vi "Nov_30 - Ramp Mode.vi"() -> ()   [LabVIEW 2020]
uses:
  <vilib>/Utility/error.llb/DialogType.ctl
  <vilib>/Analysis/3filter.llb/Filter Passband Type.ctl
  <vilib>/DAQmx/read.llb/DAQmx Read (Analog 1D DBL NChan 1Samp).vi
  <vilib>/DAQmx/create/channels.llb/DAQmx Create Channel (AI-Voltage-Basic).vi
  <vilib>/DAQmx/configure/timing.llb/DAQmx Timing (Sample Clock).vi
  <vilib>/DAQmx/miscellaneous.llb/DAQmx Fill In Error Info.vi
  <vilib>/Analysis/3filter.llb/Butterworth Filter (DBL).vi
  <vilib>/Utility/file.llb/Write Delimited Spreadsheet (string).vi
  <vilib>/Utility/file.llb/Write Delimited Spreadsheet (DBL).vi
  <vilib>/Analysis/NI_AALBase.lvlib
panel:
  out "Swing ON time":dbl
  out "Register Time":bool
  out "Swing Start Time":dbl
  out "Pre-Tension Load (N)":dbl
  out "Time To Peak (ms)":dbl
  out "Peak Value (ms)":dbl=2.0
  out "Square Wave Amp Target (N)":dbl=2.0
  in  "Auto Mode":string(combo)
  out "Release":bool
  out "Pull":bool
  in  "Working Mode":string(combo)
  out "Load Cell":dbl
  in  "Pull CMD":bool
  in  "Release CMD":bool
  out "Load Cell":dynamicdata(graph)
  in  "Motor Torque":dbl(slide) scale=0.0..5.0
  out "Swing (Consumer Loop)":bool
  in  "Master Stop":bool
  out "Consumer Loop Speed (ms)":u32
  out "Producer Loop Speed (ms)":u32
  out "Swing":bool
  out "Force Plate":dynamicdata(graph)
  out "Accelerometers":dynamicdata(graph)
  out "Enlapsed Time (sec)":dbl
  # "Motor Control"
  # "Manual"
  # "Automatic"
  # "Square"
  # "Ramp"
  # "Indicators"
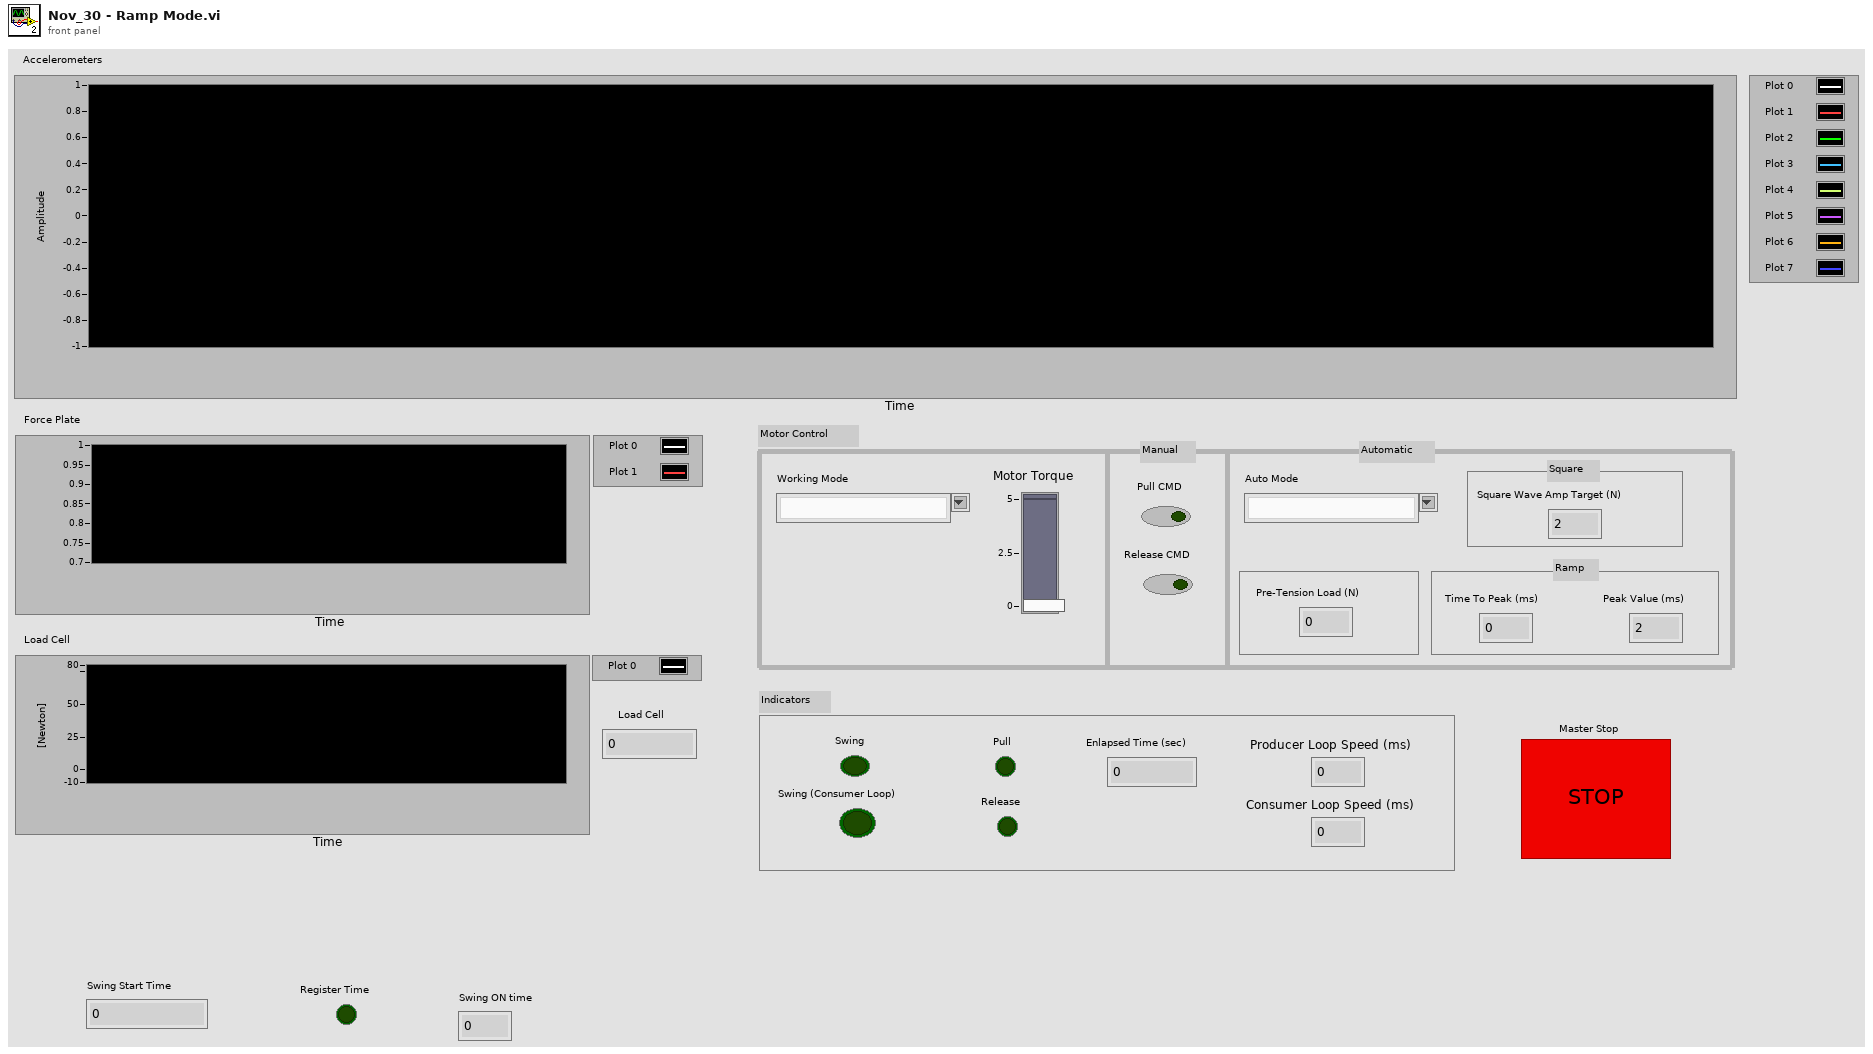
[diagram p1: front panel]
types:
  T1 = typedef "DialogType.ctl" = u16
  T2 = typedef "NI_AALBase.lvlib/Filter Passband Type.ctl" = enum32{"Lowpass", "Highpass", "Bandpass", "Bandstop"}
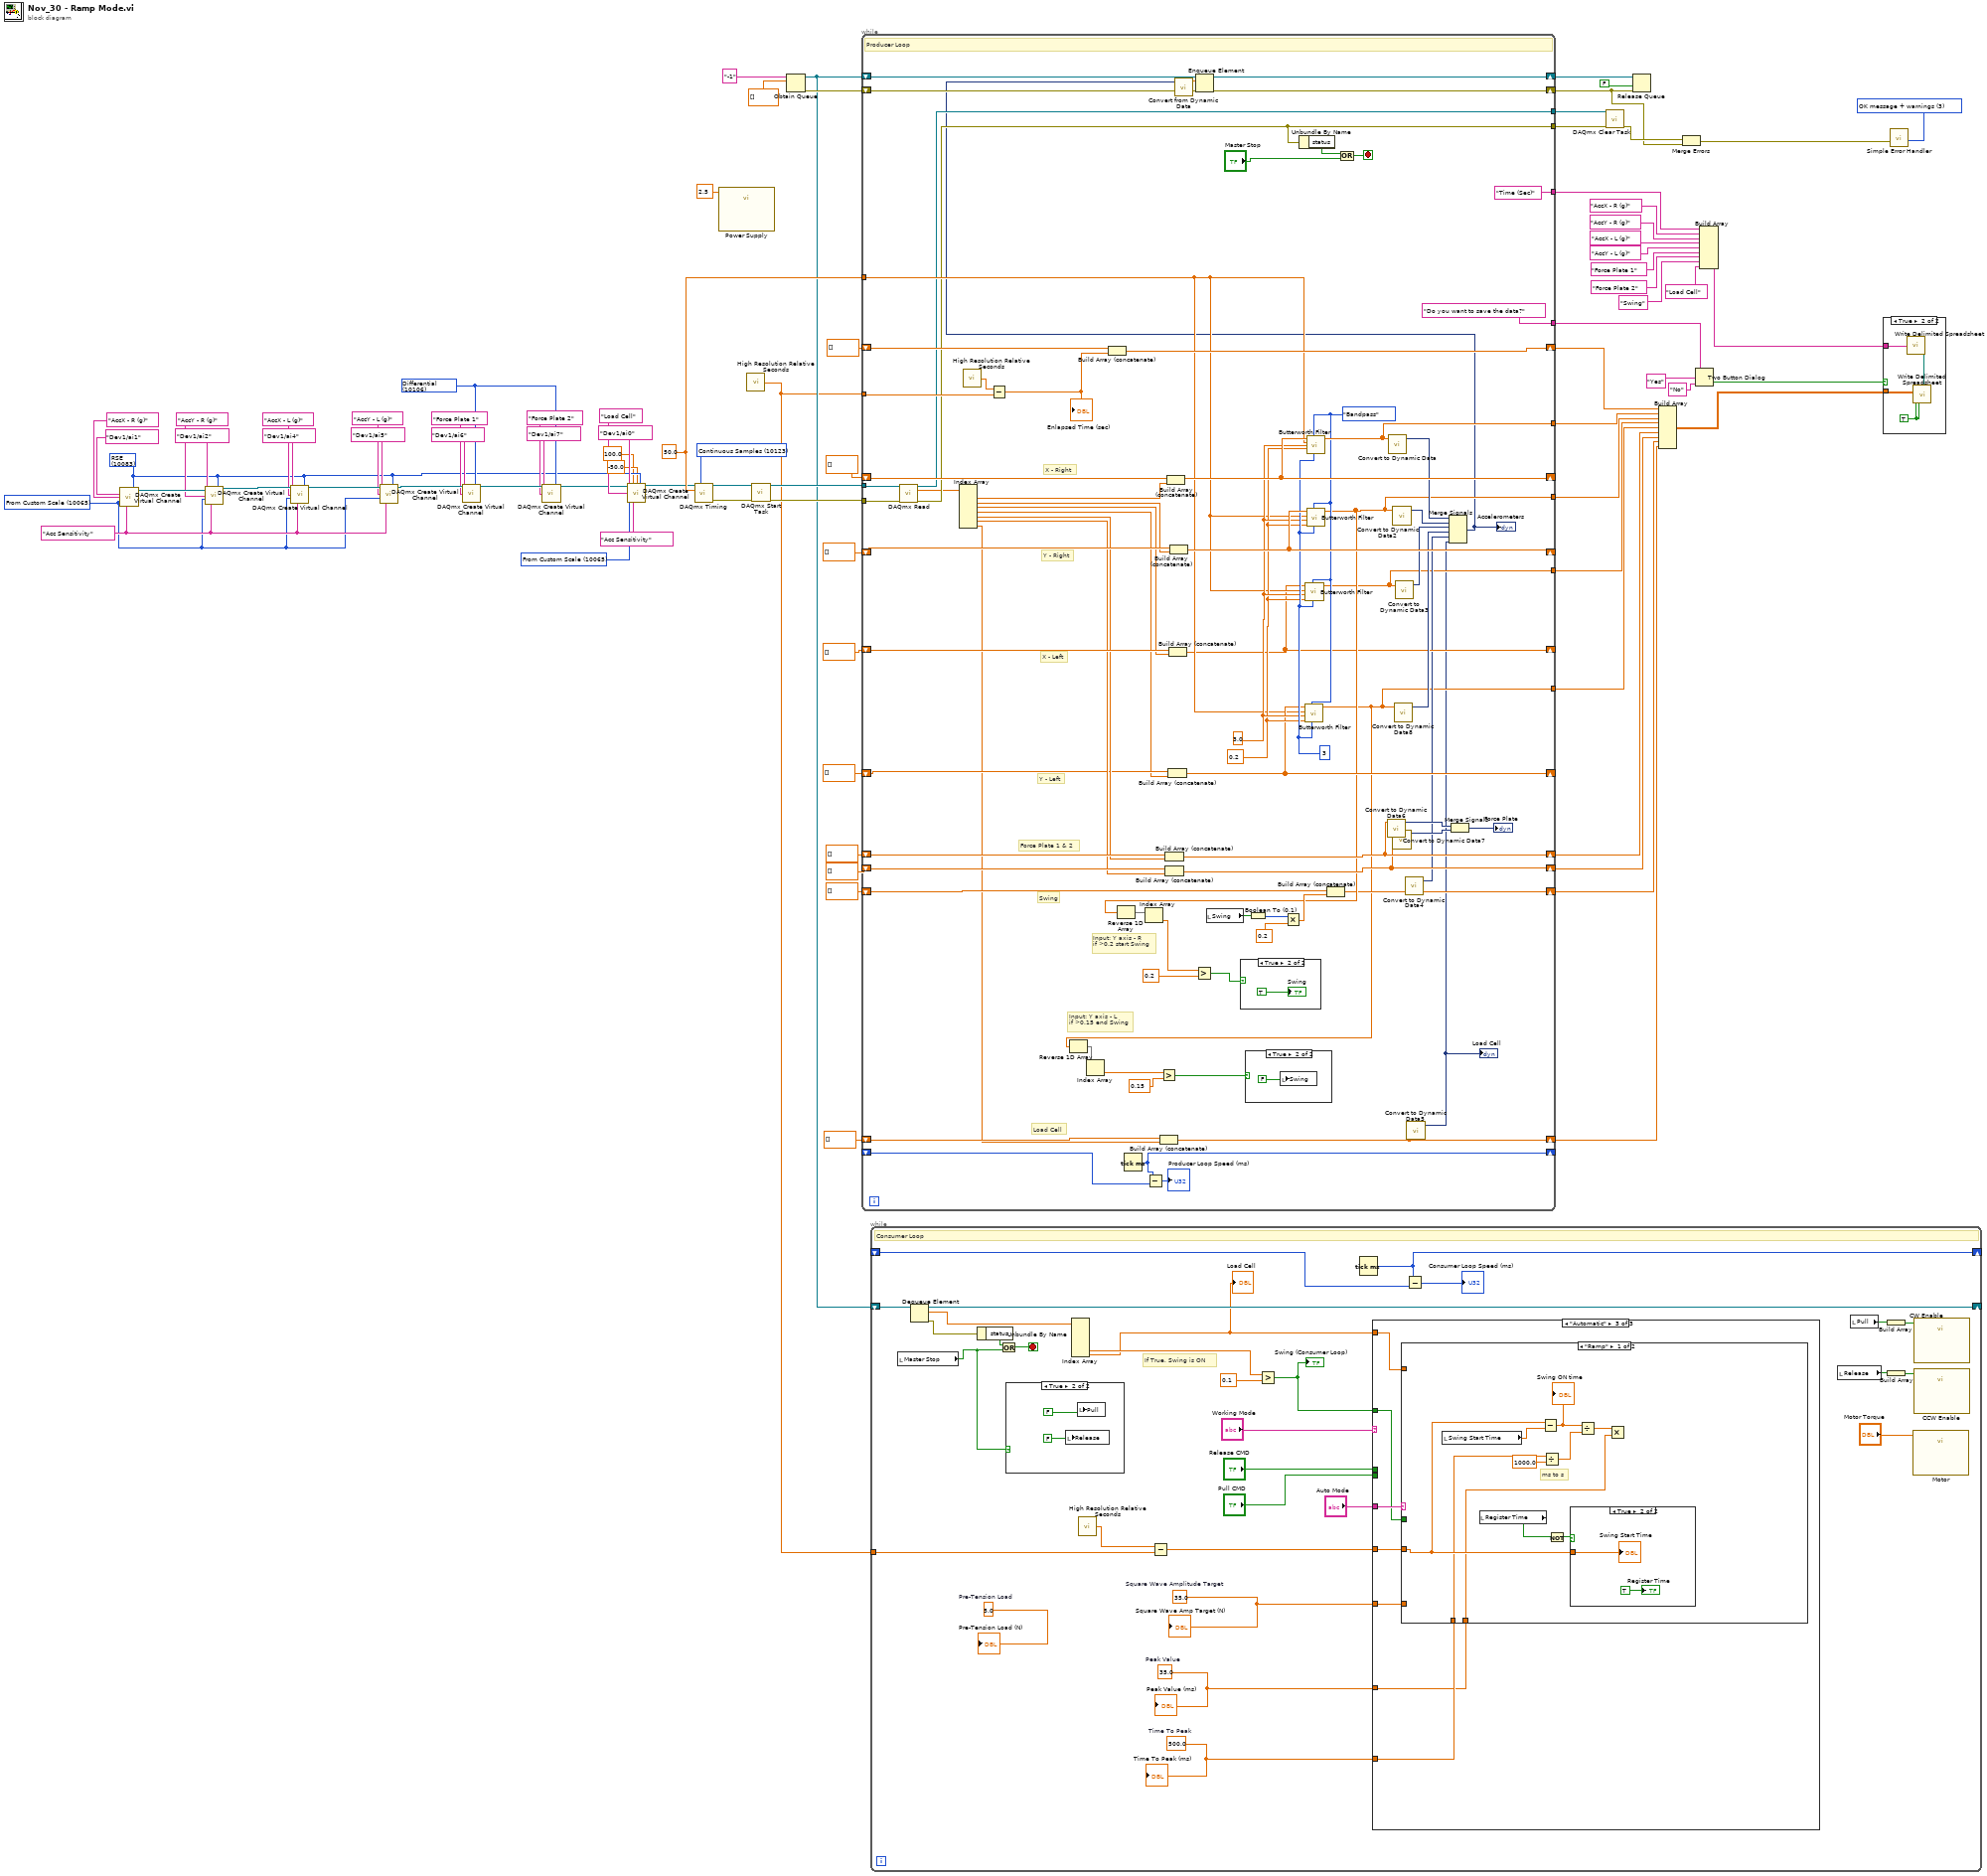
[diagram p0: block diagram]
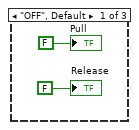
[diagram p3: hidden frame]
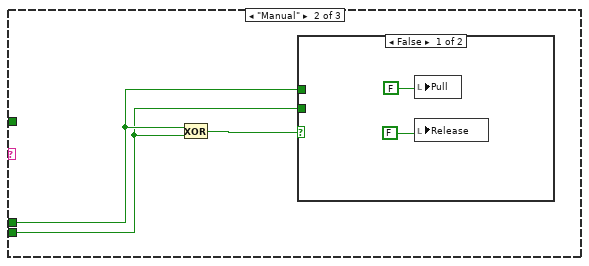
[diagram p4: hidden frame]
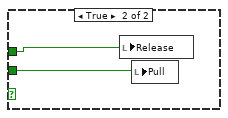
[diagram p5: hidden frame]
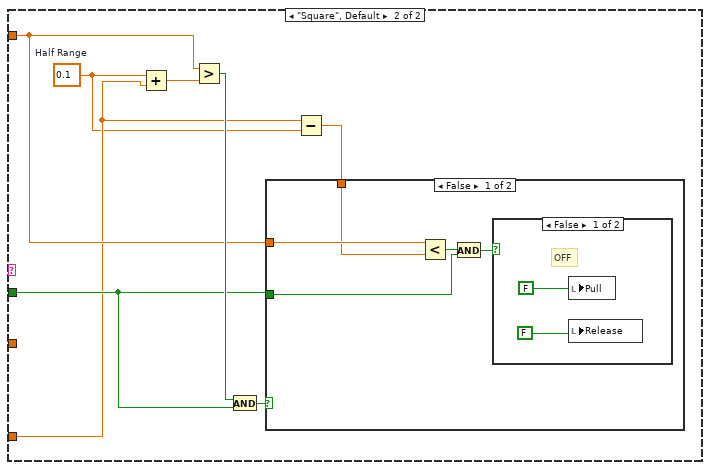
[diagram p7: hidden frame]
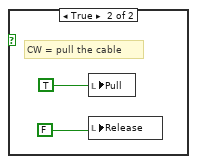
[diagram p8: hidden frame]
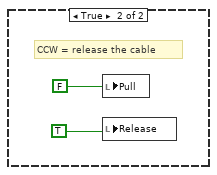
[diagram p9: hidden frame]
diagram:
  w4 = 10065 items=["Volts"=10348, "From Custom Scale"=10065] ("units")
  w20 = T1 3 items=["no dialog", "OK message", "continue or stop message", "OK message + warnings", "continue/stop + warnings"] ("type of dialog (OK msg:1)")
  w9 = 10065 items=["Volts"=10348, "From Custom Scale"=10065] ("units")
  w10 = tag "Acc Sensitivity" ("custom scale name")
  w30 = 10106 items=["Default"=-1, "RSE"=10083, "NRSE"=10078, "Differential"=10106, "Pseudodifferential"=12529] ("input terminal configuration")
  w52 = 10123 items=["Finite Samples"=10178, "Continuous Samples"=10123, "Hardware Timed Single Point"=12522] ("sample mode")
  w47 = 50.0 ("rate")
  w13 = 10083 items=["Default"=-1, "RSE"=10083, "NRSE"=10078, "Differential"=10106, "Pseudodifferential"=12529] ("input terminal configuration")
  n1 = call-poly <vilib>:"DAQmx Create Virtual Channel.vi"("input terminal configuration"=w13, "physical channels"=tag "Dev1/ai1" ("Physical channels"), "name to assign"="AccX - R (g)", "units"=w9, "custom scale name"=w10) -> ("task out"=w46:refnum<k21>)  [unwired: 9 in, 1 out]
  n2 = call-poly <vilib>:"DAQmx Create Virtual Channel.vi"("task in"=w46, "input terminal configuration"=w13, "physical channels"=tag "Dev1/ai2", "name to assign"="AccY - R (g)", "units"=w9, "custom scale name"=w10) -> ("task out"=w45:refnum<k21>)  [unwired: 8 in, 1 out]
  n3 = call-poly <vilib>:"DAQmx Create Virtual Channel.vi"("task in"=w45, "input terminal configuration"=w13, "physical channels"=tag "Dev1/ai4", "name to assign"="AccX - L (g)", "units"=w9, "custom scale name"=w10) -> ("task out"=w44:refnum<k21>)  [unwired: 8 in, 1 out]
  n4 = call-poly <vilib>:"DAQmx Create Virtual Channel.vi"("task in"=w44, "input terminal configuration"=w13, "physical channels"=tag "Dev1/ai5", "name to assign"="AccY - L (g)", "units"=w9, "custom scale name"=w10) -> ("task out"=w43:refnum<k21>)  [unwired: 8 in, 1 out]
  n5 = call-poly <vilib>:"DAQmx Create Virtual Channel.vi"("task in"=w43, "input terminal configuration"=w30, "physical channels"=tag "Dev1/ai6", "name to assign"="Force Plate 1" ("element")) -> ("task out"=w37:refnum<k21>)  [unwired: 10 in, 1 out]
  n6 = call-poly <vilib>:"DAQmx Create Virtual Channel.vi"("task in"=w37, "input terminal configuration"=w30, "physical channels"=tag "Dev1/ai7", "name to assign"="Force Plate 2" ("element")) -> ("task out"=w12:refnum<k21>)  [unwired: 10 in, 1 out]
  n7 = call-poly <vilib>:"DAQmx Create Virtual Channel.vi"("task in"=w12, "maximum value"=100.0, "minimum value"=-50.0, "input terminal configuration"=w13, "physical channels"=tag "Dev1/ai0", "name to assign"="Load Cell", "units"=w4, "custom scale name"=tag "Acc Sensitivity") -> ("task out"=w11:refnum<k21>)  [unwired: 6 in, 1 out]
  n8 = call-poly <vilib>:"DAQmx Timing.vi"("task/channels in"=w11, "sample mode"=w52, "rate"=w47) -> ("task out"=w51:refnum<k21>, "error out"=w50:errorcluster)  [unwired: 11 in]
  n9 = call "Power Supply"("data"=2.5) -> ()  [unwired: 17 in, 2 out]
  n10 = call <vilib>:"High Resolution Relative Seconds.vi"() -> ("relative seconds"=w1:dbl)
  n11 = call <vilib>:"DAQmx Start Task.vi"("task/channels in"=w51, "error in"=w50) -> ("task out"=w49:refnum<k21>, "error out"=w48:errorcluster)  [unwired: 12 in]
  n12 = Obtain Queue(name (unnamed)="-1", element data type=dbl[] []) -> (queue out=w16:refnum<queue>, error out=w25:errorcluster)  [unwired: 3 in, 1 out]
  n13 = while {
    tunnel: w49 -> [w159]
    tunnel: w48 -> [w158]
    tunnel: w1 -> [w156]
    shift-right: [w140] -> w80
    shift-left: dbl[] [] -> [w154]
    shift-right: [w144] -> _
    shift-left: dbl[] [] -> [w153]
    shift-right: [w143] -> _
    shift-left: dbl[] [] -> [w152]
    tunnel: ["Time (Sec)"] -> w55
    tunnel: ["Do you want to save the data?" ("message")] -> w72
    shift-right: [w104] -> w59
    shift-left: dbl[] [] -> [w149]
    shift-right: [w105] -> _
    shift-left: dbl[] [] -> [w141]
    shift-right: [w130] -> w57
    shift-left: dbl[] [] -> [w133]
    shift-right: [w128] -> w58
    shift-left: dbl[] [] -> [w132]
    tunnel: [w126] -> w62
    tunnel: [w108] -> w61
    tunnel: [w100] -> w60
    shift-right: [w119] -> _
    shift-left: dbl[] [] -> [w118]
    tunnel: [w99] -> w56
    tunnel: w47 -> [w116]
    shift-right: [w110] -> _
    shift-left: _ -> [w109]
    shift-right: [w93] -> w24
    shift-left: w16 -> [w94]
    shift-right: [w91] -> w17
    shift-left: w25 -> [w92]
    tunnel: [w98] -> w22
    tunnel: [w95] -> w21
    shift-right: [w86] -> w7
    shift-left: dbl[] [] -> [w85]
    stop <- w96 stop-if-true
    w123 = 3 ("order")
    w121 = 0.2 ("low cutoff freq: fl")
    w122 = 3.0 ("high cutoff freq: fh")
    w117 = Filter_Passband_Type."Bandpass" ("filter type")
    # "X - Right"
    # "Y - Right"
    # "X - Left"
    # "Y - Left"
    # "Force Plate 1 & 2"
    # "Swing"
    # "Load Cell"
    # "Input: Y axis - L\nif >0.15 end Swing"
    # "Input: Y axis - R\nif >0.2 start Swing"
    # "Producer Loop"
    n14 = call-poly <vilib>:"DAQmx Read.vi"("task/channels in"=w159, "error in"=w158) -> ("task out"=w98:refnum<k21>, "data"=w90:dbl[], "error out"=w95:errorcluster)  [unwired: 11 in]
    n15 = Index Array(array=w90) -> (element #1=w115:dbl, element #2=w114:dbl, element #3=w113:dbl, element #4=w112:dbl, element #5=w124:dbl, element #6=w125:dbl, element #7=w84:dbl)  [unwired: 7 in]
    n16 = call <vilib>:"High Resolution Relative Seconds.vi"() -> ("relative seconds"=w157:dbl)
    n17 = Subtract(x=w157, y=w156) -> (x-y=w155:dbl)
    "Enlapsed Time (sec)" <- w155
    n18 = Build Array (concatenate)(w154, w155) -> (w140:dbl[])
    n19 = Tick Count (ms)() -> (millisecond timer value=w110:u32)
    n20 = Subtract(x=w110, y=w109) -> (x-y=→"Producer Loop Speed (ms)":u32)
    n21 = Build Array (concatenate)(w85, w84) -> (w86:dbl[])
    n22 = Build Array (concatenate)(w133, w124) -> (w130:dbl[])
    n23 = Build Array (concatenate)(w132, w125) -> (w128:dbl[])
    n24 = Build Array (concatenate)(w153, w115) -> (w144:dbl[])
    n25 = Build Array (concatenate)(w118, w112) -> (w119:dbl[])
    n26 = Build Array (concatenate)(w141, w113) -> (w105:dbl[])
    n27 = Build Array (concatenate)(w152, w114) -> (w143:dbl[])
    n28 = local read "Swing"() -> (w142:bool)
    n29 = Boolean To (0,1)(Boolean=w142) -> (0, 1=w147:i16)
    n30 = Multiply(x=w147, y=0.2) -> (x*y=w148:dbl)
    n31 = Unbundle By Name(w95) -> ("status"=w97:bool)
    n32 = call-poly <vilib>:"Butterworth Filter.vi"("order"=w123, "filter type"=w117, "low cutoff freq: fl"=w121, "high cutoff freq: fh"=w122, "sampling freq: fs"=w116, "X"=w119) -> ("Filtered X"=w99:dbl[])  [unwired: 2 in, 1 out]
    n33 = Reverse 1D Array(array=w99) -> (reversed array=w135:dbl[])
    n34 = Index Array(array=w135) -> (element=w134:dbl)  [unwired: 1 in]
    n35 = Greater?(x=w134, y=0.15) -> (0:w102:bool)
    n36 = case shown="True" w102 {
      frame False {
      }
      frame True {
        n37 = local write "Swing"(FALSE) -> ()
      }
    }
    n38 = call-poly <vilib>:"Butterworth Filter.vi"("order"=w123, "filter type"=w117, "low cutoff freq: fl"=w121, "high cutoff freq: fh"=w122, "sampling freq: fs"=w116, "X"=w105) -> ("Filtered X"=w100:dbl[])  [unwired: 2 in, 1 out]
    n39 = call-poly <vilib>:"Butterworth Filter.vi"("order"=w123, "filter type"=w117, "low cutoff freq: fl"=w121, "high cutoff freq: fh"=w122, "sampling freq: fs"=w116, "X"=w144) -> ("Filtered X"=w126:dbl[])  [unwired: 2 in, 1 out]
    n40 = call-poly <vilib>:"Butterworth Filter.vi"("order"=w123, "filter type"=w117, "low cutoff freq: fl"=w121, "high cutoff freq: fh"=w122, "sampling freq: fs"=w116, "X"=w143) -> ("Filtered X"=w108:dbl[])  [unwired: 2 in, 1 out]
    n41 = Reverse 1D Array(array=w108) -> (reversed array=w145:dbl[])
    n42 = Index Array(array=w145) -> (element=w107:dbl)  [unwired: 1 in]
    n43 = Greater?(x=w107, y=0.2) -> (0:w101:bool)
    n44 = case shown="True" w101 {
      frame False {
      }
      frame True {
        "Swing" <- TRUE
      }
    }
    n45 = Build Array (concatenate)(w149, w148) -> (w104:dbl[])
    n46 = Or(x=w97, y="Master Stop") -> (x .or. y?=w96:bool)
    n47 = call "Convert to Dynamic Data6"("Array"=w130) -> ("Dynamic Data Type"=w129:dynamicdata)  [unwired: 3 in]
    n48 = call "Convert to Dynamic Data"("Array"=w126) -> ("Dynamic Data Type"=w139:dynamicdata)  [unwired: 3 in]
    n49 = call "Convert to Dynamic Data2"("Array"=w108) -> ("Dynamic Data Type"=w138:dynamicdata)  [unwired: 3 in]
    n50 = call "Convert to Dynamic Data7"("Array"=w128) -> ("Dynamic Data Type"=w127:dynamicdata)  [unwired: 3 in]
    n51 = call "Convert to Dynamic Data8"("Array"=w99) -> ("Dynamic Data Type"=w120:dynamicdata)  [unwired: 3 in]
    n52 = call "Convert to Dynamic Data3"("Array"=w100) -> ("Dynamic Data Type"=w137:dynamicdata)  [unwired: 3 in]
    n53 = call "Convert to Dynamic Data4"("Array"=w104) -> ("Dynamic Data Type"=w103:dynamicdata)  [unwired: 3 in]
    n54 = call "Convert to Dynamic Data5"("Array"=w86) -> ("Dynamic Data Type"=w83:dynamicdata)  [unwired: 3 in]
    "Load Cell" <- w83
    n55 = Merge Signals(w139, w138, w137, w120, w103, w83) -> (w88:dynamicdata)
    "Accelerometers" <- w88
    n56 = call "Convert from Dynamic Data"("Dynamic Data Type"=w88) -> ("Array"=w87:dbl[])  [unwired: 3 in]
    n57 = Enqueue Element(queue=w94, element=w87, error in (no error)=w92) -> (queue out=w93:refnum<queue>, error out=w91:errorcluster)  [unwired: 1 in, 1 out]
    n58 = Merge Signals(w129, w127) -> (→"Force Plate":dynamicdata)
  }
  n59 = while {
    shift-right: [w190] -> _
    shift-left: w16 -> [w191]
    shift-right: [w187] -> _
    shift-left: _ -> [w188]
    tunnel: w1 -> [w163]
    stop <- w185 stop-if-true
    w165 = 5.0  # Pre-Tension Load
    w166 = 500.0  # Time To Peak
    w167 = 35.0  # Peak Value
    w168 = 35.0  # Square Wave Amplitude Target
    # "If True, Swing is ON"
    # "Consumer Loop"
    n60 = local read "Master Stop"() -> (w170:bool)
    n61 = Dequeue Element(queue=w191) -> (queue out=w190:refnum<queue>, element=w183:dbl[], error out=w184:errorcluster)  [unwired: 2 in, 1 out]
    n62 = Unbundle By Name(w184) -> ("status"=w186:bool)
    n63 = Or(x=w186, y=w170) -> (x .or. y?=w185:bool)
    n64 = case shown="True" w170 {
      frame False {
      }
      frame True {
        n65 = local write "Release"(FALSE) -> ()
        n66 = local write "Pull"(FALSE) -> ()
      }
    }
    n67 = Index Array(array=w183) -> (element #5=w182:dbl, element #6=w180:dbl)  [unwired: 6 in, 4 out]
    "Load Cell" <- w180
    n68 = call <vilib>:"High Resolution Relative Seconds.vi"() -> ("relative seconds"=w164:dbl)
    n69 = Subtract(x=w164, y=w163) -> (x-y=w162:dbl)
    n70 = Greater?(x=w182, y=0.1) -> (0:w171:bool)
    "Swing (Consumer Loop)" <- w171
    n71 = Tick Count (ms)() -> (millisecond timer value=w187:u32)
    n72 = case shown="\"Automatic\"" "Working Mode" {
      tunnel: w180 -> [_ _ w207]
      tunnel: "Release CMD" -> [_ w197 _]
      tunnel: "Pull CMD" -> [_ w196 _]
      tunnel: w171 -> [_ _ w208]
      tunnel: "Auto Mode" -> [_ _ w209]
      tunnel: w168 -> [_ _ w206]
      tunnel: w167 -> [_ _ w203]
      tunnel: w166 -> [_ _ w204]
      tunnel: w162 -> [_ _ w205]
      frame "OFF", Default {
        "Pull" <- FALSE
        "Release" <- FALSE
      }
      frame "Manual" {
        n73 = Exclusive Or(1:w196, 2:w197) -> (0:w198:bool)
        n74 = case shown="False" w198 {
          tunnel: w197 -> [_ w201]
          tunnel: w196 -> [_ w202]
          frame False {
            n75 = local write "Pull"(FALSE) -> ()
            n76 = local write "Release"(FALSE) -> ()
          }
          frame True {
            n77 = local write "Release"(w201) -> ()
            n78 = local write "Pull"(w202) -> ()
          }
        }
      }
      frame "Automatic" {
        n79 = case shown="\"Ramp\"" w209 {
          tunnel: w208 -> [_ w227]
          tunnel: w207 -> [_ w226]
          tunnel: w206 -> [_ w223]
          tunnel: w205 -> [w218 _]
          tunnel: w204 -> [w214 _]
          tunnel: w203 -> [w210 _]
          frame "Ramp" {
            # "ms to s"
            n80 = local read "Swing Start Time"() -> (w217:dbl)
            n81 = local read "Register Time"() -> (w219:bool)
            n82 = Subtract(x=w218, y=w217) -> (x-y=w215:dbl)
            "Swing ON time" <- w215
            n83 = Divide(x=w214, y=1000.0) -> (x/y=w212:dbl)
            n84 = Not(x=w219) -> (.not. x?=w216:bool)
            n85 = case shown="True" w216 {
              tunnel: w218 -> [_ w221]
              frame False {
              }
              frame True {
                "Swing Start Time" <- w221
                "Register Time" <- TRUE
              }
            }
            n86 = Divide(x=w215, y=w212) -> (x/y=w211:dbl)
            n87 = Multiply(x=w211, y=w210) -> ()  [unwired: 1 out]
          }
          frame "Square", Default {
            w222 = 0.1  # Half Range
            n88 = Add(x=w222, y=w223) -> (x+y=w225:dbl)
            n89 = Greater?(x=w226, y=w225) -> (0:w229:bool)
            n90 = And(x=w229, y=w227) -> (x .and. y?=w228:bool)
            n91 = Subtract(x=w223, y=w222) -> (x-y=w224:dbl)
            n92 = case shown="False" w228 {
              tunnel: w226 -> [w234 _]
              tunnel: w227 -> [w231 _]
              tunnel: w224 -> [w230 _]
              frame False {
                n93 = Less?(x=w234, y=w230) -> (x < y?=w232:bool)
                n94 = And(x=w232, y=w231) -> (x .and. y?=w233:bool)
                n95 = case shown="False" w233 {
                  frame False {
                    # "OFF"
                    n96 = local write "Pull"(FALSE) -> ()
                    n97 = local write "Release"(FALSE) -> ()
                  }
                  frame True {
                    # "CW = pull the cable"
                    n98 = local write "Pull"(TRUE) -> ()
                    n99 = local write "Release"(FALSE) -> ()
                  }
                }
              }
              frame True {
                # "CCW = release the cable"
                n100 = local write "Pull"(FALSE) -> ()
                n101 = local write "Release"(TRUE) -> ()
              }
            }
          }
        }
      }
    }
    n102 = Subtract(x=w187, y=w188) -> (x-y=→"Consumer Loop Speed (ms)":u32)
    n103 = local read "Release"() -> (w174:bool)
    n104 = local read "Pull"() -> (w175:bool)
    n105 = Build Array(w175) -> (w177:bool[])
    n106 = Build Array(w174) -> (w176:bool[])
    n107 = call "Motor"("data"="Motor Torque") -> ()  [unwired: 17 in, 2 out]
    n108 = call "CW Enable"("data"=w177) -> ()  [unwired: 17 in, 2 out]
    n109 = call "CCW Enable"("data"=w176) -> ()  [unwired: 17 in, 2 out]
    "Square Wave Amp Target (N)" <- w168
    "Peak Value (ms)" <- w167
    "Time To Peak (ms)" <- w166
    "Pre-Tension Load (N)" <- w165
  }
  n110 = call <vilib>:"DAQmx Clear Task.vi"("task in"=w22, "error in"=w21) -> ("error out"=w18:errorcluster)  [unwired: 13 out]
  n111 = Release Queue(queue=w24, force destroy? (F)=FALSE, error in (no error)=w17) -> ()  [unwired: 3 out]
  n112 = Build Array(w80, w62, w61, w60, w56, w57, w58, w59, w7) -> (w79:dbl[][])
  n113 = Merge Errors(w18, w17) -> (w19:errorcluster)
  n114 = Two Button Dialog(message=w72, 1:"No" ("F button name (\"Cancel\")"), 2:"Yes" ("T button name (\"OK\")")) -> (T button?=w75:bool)
  n115 = Build Array(w55, "AccX - R (g)", "AccY - R (g)", "AccX - L (g)", "AccY - L (g)", "Force Plate 1" ("element"), "Force Plate 2" ("element"), "Swing" ("element"), "Load Cell" ("element")) -> (w78:string[])
  n116 = case shown="True" w75 {
    tunnel: w79 -> [_ w244]
    tunnel: w78 -> [_ w243]
    frame False {
    }
    frame True {
      w242 = TRUE ("transpose? (no:F)")
      n117 = call-poly <vilib>:"Write Delimited Spreadsheet.vi"("1D data"=w243) -> ("new file path (Not A Path if cancelled)"=w241:path)  [unwired: 13 in, 1 out]
      n118 = call-poly <vilib>:"Write Delimited Spreadsheet.vi"("file path (dialog if empty)"=w241, "2D data"=w244, "append to file? (new file:F)"=w242, "transpose? (no:F)"=w242) -> ()  [unwired: 10 in, 2 out]
    }
  }
  n119 = call <vilib>:"Simple Error Handler.vi"("type of dialog (OK msg:1)"=w20, "error in (no error)"=w19) -> ()  [unwired: 8 out]
